vi "dfd_Quantize Filter.vi"(8 "error in (no error)":errorcluster, 11 "filter in":T1={"mSRate_Fs"=1.0, "mSRate_Version"="1.0", "mSRate_Comments"="", "mSRate_OrgCoef"={"type"=enum."Undefined", "gain"=1.0, "coef a (k)"=[], "coef b (v)"=[]}, "mSRate_CurCoef"={"type"=enum."Undefined", "gain"=1.0, "coef a (k)"=[], "coef b (v)"=[]}, "mSRate_Quantized?"=FALSE, "mSRate_QCoef"={"type"=enum."Undefined", "gain"=1.0, "coef a (k)"=[], "coef b (v)"=[]}, "mSRate_QSettings"=[], "mSRate_Order"=0, "mSRate_Scaling"={"mSRate_ScaleByPowerOf2?"=FALSE, "mSRate_ScaleType"=enum."No Norm"}} {"mSRate_QSettings"."source" items=["Coef a/k"=0, "Coef b/v"=7, "Input"=1, "Output"=2, "Multiplicand"=3, "Product"=4, "Sum"=5, "Delay"=6, "Gain"=8]}) -> (0 "error out":errorcluster, 3 "filter out":T1={"mSRate_Fs"=1.0, "mSRate_Version"="1.0", "mSRate_Comments"="", "mSRate_OrgCoef"={"type"=enum."Undefined", "gain"=1.0, "coef a (k)"=[], "coef b (v)"=[]}, "mSRate_CurCoef"={"type"=enum."Undefined", "gain"=1.0, "coef a (k)"=[], "coef b (v)"=[]}, "mSRate_Quantized?"=FALSE, "mSRate_QCoef"={"type"=enum."Undefined", "gain"=1.0, "coef a (k)"=[], "coef b (v)"=[]}, "mSRate_QSettings"=[], "mSRate_Order"=0, "mSRate_Scaling"={"mSRate_ScaleByPowerOf2?"=FALSE, "mSRate_ScaleType"=enum."No Norm"}} {"mSRate_QSettings"."source" items=["Coef a/k"=0, "Coef b/v"=7, "Input"=1, "Output"=2, "Multiplicand"=3, "Product"=4, "Sum"=5, "Delay"=6, "Gain"=8]})   [LabVIEW 2017, in "NI_DigFilter_FXP.lvlib"]
uses:
  <vilib>/addons/Digital Filter Design/NI_DigFilter_FXP.lvlib
  <vilib>/addons/Digital Filter Design/_Objects.llb/DFD Filter Obj.ctl
  <vilib>/addons/Digital Filter Design/_Objects.llb/DFD Filter Coef.ctl
  <vilib>/addons/Digital Filter Design/_Objects.llb/DFD Filter Structure Type Selector.ctl
  <vilib>/addons/Digital Filter Design/_Objects.llb/dfd_Internal Quantization Settings.ctl
  <vilib>/addons/Digital Filter Design/_Objects.llb/dfd_Internal Quantization Srcs.ctl
  <vilib>/addons/Digital Filter Design/_Objects.llb/DFD Coef Norm Type.ctl
  <vilib>/addons/Digital Filter Design/FXPLib.llb/dfd_FXP Casting (scaler).vi
  <vilib>/addons/Digital Filter Design/FXPLib.llb/dfd_FXP Casting (vector).vi
  <vilib>/addons/Digital Filter Design/NI_DigFilterLicensed.lvlib
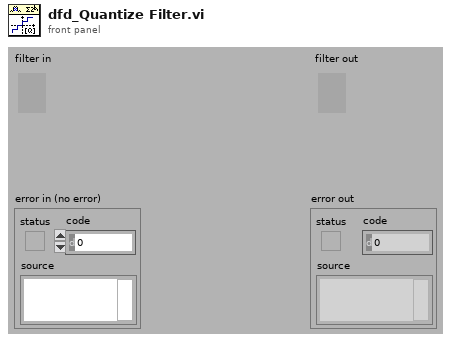
[diagram p1: front panel]
types:
  T1 = typedef "NI_DigFilterLicensed.lvlib/DFD Filter Obj.ctl" = cluster{"mSRate_Fs":dbl, "mSRate_Version":string, "mSRate_Comments":string, "mSRate_OrgCoef":T2, "mSRate_CurCoef":T2, "mSRate_Quantized?":bool, "mSRate_QCoef":T2, "mSRate_QSettings":T4[], "mSRate_Order":i32, "mSRate_Scaling":cluster{"mSRate_ScaleByPowerOf2?":bool, "mSRate_ScaleType":T6}}
  T2 = typedef "NI_DigFilterLicensed.lvlib/DFD Filter Coef.ctl" = cluster{"type":T3, "gain":dbl, "coef a (k)":dbl[], "coef b (v)":dbl[]}
  T3 = typedef "NI_DigFilterLicensed.lvlib/DFD Filter Structure Type Selector.ctl" = enum16{"Undefined", "FIR Direct Form", "FIR Direct Form Transposed", "FIR Symmetric", "FIR Antisymmetric", "IIR Direct Form I", "IIR Direct Form I Transposed", "IIR Direct Form II", "IIR Direct Form II Transposed", "IIR Cascaded Second Order Sections Form I", "IIR Cascaded Second Order Sections Form I Transposed", "IIR Cascaded Second Order Sections Form II", "IIR Cascaded Second Order Sections Form II Transposed", "Lattice Allpass (basic sections)", "Lattice Allpass (one multiplier sections)", "Lattice Allpass (normalized sections)", "Lattice AR (basic sections)", "Lattice AR (one multiplier sections)", "Lattice AR (normalized sections)", "Lattice MA (minimum phase)", "Lattice MA (maximum phase)", "Lattice ARMA (basic sections)", "Lattice ARMA (one multiplier sections)", "Lattice ARMA (normalized sections)"}
  T4 = typedef "NI_DigFilterLicensed.lvlib/dfd_Internal Quantization Settings.ctl" = cluster{"source":T5, "wl":i16, "iwl":i16, "overflow mode":enum16{"Saturation", "Wrap"}, "rounding mode":enum16{"Nearest", "Truncation"}, "signed?":bool}
  T5 = typedef "NI_DigFilterLicensed.lvlib/dfd_Internal Quantization Srcs.ctl" = u16
  T6 = typedef "NI_DigFilterLicensed.lvlib/DFD Coef Norm Type.ctl" = enum16{"No Norm", "Time Domain 1-Norm", "Time Domain 2-Norm", "Time Domain Inf-Norm"}
  T7 = typedef "NI_DigFilterLicensed.lvlib/DFD Filter Structure Id.ctl" = enum16{"Undefined", "FIR", "IIR Direct", "IIR SOS", "IIR Allpass", "IIR AR", "IIR ARMA"}
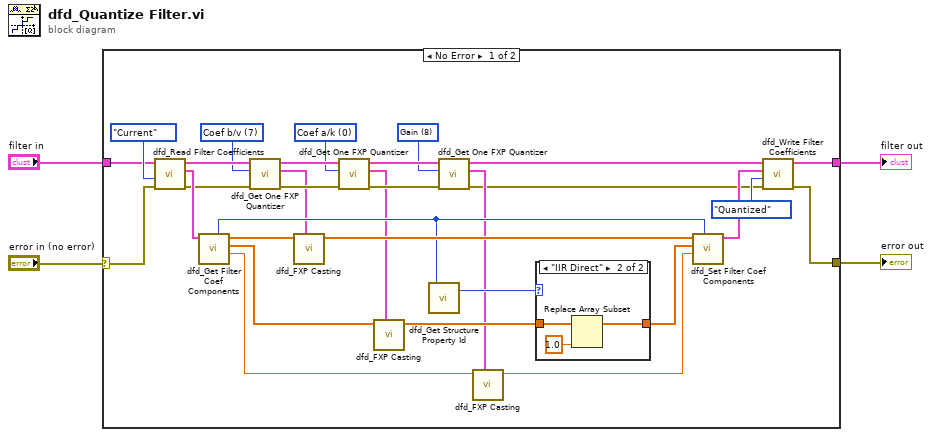
[diagram p0: block diagram]
diagram:
  n1 = case shown="No Error" "error in (no error)" {
    selector: "error in (no error)" -> [w7 w41]
    tunnel: "filter in" -> [w25 w40]
    tunnel: [w6 w41] -> w1
    tunnel: [w5 w40] -> w2
    frame No Error {
      w17 = T5 8 items=["Coef a/k"=0, "Coef b/v"=7, "Input"=1, "Output"=2, "Multiplicand"=3, "Product"=4, "Sum"=5, "Delay"=6, "Gain"=8] ("quantization source")
      w19 = T5 0 items=["Coef a/k"=0, "Coef b/v"=7, "Input"=1, "Output"=2, "Multiplicand"=3, "Product"=4, "Sum"=5, "Delay"=6, "Gain"=8] ("quantization source")
      w22 = T5 7 items=["Coef a/k"=0, "Coef b/v"=7, "Input"=1, "Output"=2, "Multiplicand"=3, "Product"=4, "Sum"=5, "Delay"=6, "Gain"=8] ("quantization source")
      n2 = call <vilib>:"dfd_Read Filter Coefficients.vi"("error in (no error)"=w7, "coef source"=enum16{"Original", "Current", "Quantized"}."Current", "filter in"=w25) -> ("error out"=w21:errorcluster, "filter coef"=w34:T2, "filter out"=w24:T1)  [unwired: 6 out]
      n3 = call <vilib>:"dfd_Get Filter Coef Components.vi"("filter coef"=w34) -> ("gain"=w12:dbl, "coef a (k)"=w32:dbl[], "coef b (v)"=w33:dbl[], "type"=w23:T3)  [unwired: 1 in, 6 out]
      n4 = call <vilib>:"dfd_Get One FXP Quantizer.vi"("error in (no error)"=w21, "quantization source"=w22, "filter in"=w24) -> ("error out"=w16:errorcluster, "quantization settings"=w14:T4, "filter out"=w20:T1)  [unwired: 6 out]
      n5 = call-poly <vilib>:"dfd_FXP Casting.vi"("quantization settings"=w14, "values in"=w33) -> ("values out"=w31:dbl[])  [unwired: 1 in, 6 out]
      n6 = call <vilib>:"dfd_Get One FXP Quantizer.vi"("error in (no error)"=w16, "quantization source"=w19, "filter in"=w20) -> ("error out"=w15:errorcluster, "quantization settings"=w13:T4, "filter out"=w18:T1)  [unwired: 6 out]
      n7 = call-poly <vilib>:"dfd_FXP Casting.vi"("quantization settings"=w13, "values in"=w32) -> ("values out"=w27:dbl[])  [unwired: 1 in, 6 out]
      n8 = call <vilib>:"dfd_Get Structure Property Id.vi"("structure type"=w23) -> ("filter structure id"=w28:T7)  [unwired: 1 out]
      n9 = call <vilib>:"dfd_Get One FXP Quantizer.vi"("error in (no error)"=w15, "quantization source"=w17, "filter in"=w18) -> ("error out"=w9:errorcluster, "quantization settings"=w11:T4, "filter out"=w8:T1)  [unwired: 6 out]
      n10 = call-poly <vilib>:"dfd_FXP Casting.vi"("quantization settings"=w11, "value in"=w12) -> ("value out"=w10:dbl)  [unwired: 1 in, 6 out]
      n11 = case shown="\"IIR Direct\"" w28 {
        tunnel: w27 -> [w36 w39]
        tunnel: [w36 w37] -> w26
        frame "Undefined", Default {
        }
        frame "IIR Direct" {
          n12 = Replace Array Subset(array=w39, new element=1.0 ("new element/subarray")) -> (w37:dbl[])  [unwired: 1 in]
        }
      }
      n13 = call <vilib>:"dfd_Set Filter Coef Components.vi"("type"=w23, "gain"=w10, "coef a (k)"=w26, "coef b (v)"=w31) -> ("filter coef"=w29:T2)  [unwired: 1 in, 6 out]
      n14 = call <vilib>:"dfd_Write Filter Coefficients.vi"("error in (no error)"=w9, "coef source"=enum16{"Original", "Current", "Quantized"}."Quantized", "filter coef"=w29, "filter in"=w8) -> ("error out"=w6:errorcluster, "filter out"=w5:T1)  [unwired: 6 out]
    }
    frame Error {
    }
  }
  "filter out" <- w2
  "error out" <- w1
